vi "PathAtTicket.vi"(0 "Ticket Name":string) -> (8 "path":path)   [LabVIEW 2021]
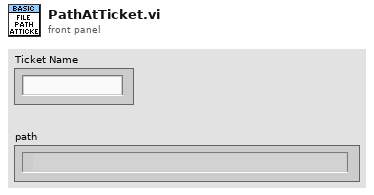
[diagram p1: front panel]
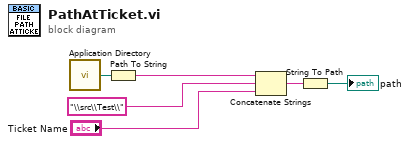
[diagram p0: block diagram]
diagram:
  n1 = call <vilib>:"Application Directory.vi"() -> ("Application Directory"=w6:path)
  n2 = Path To String(path=w6) -> (string=w1:string)
  n3 = Concatenate Strings(w1, "\\src\\Test\\" ("string"), "Ticket Name") -> (w4:string)
  n4 = String To Path(string=w4) -> (path=→"path":path)
